vi "Main.vi"() -> ()   [LabVIEW 2020]
doc: "Use this template to build a user interface event handler design pattern. Use this pattern for dialog boxes and other user interfaces. You also can create and execute user-defined events that the VI can handle the same way as user interface events."
uses:
  45491af6-0a4f-43f3-a96b-97e2b64ce829.vi
  87b3b347-8260-4ce2-8b38-5772d22dc736.vi
  421a8988-43c2-4a9a-bdb3-95a91e2f1d3f.vi
  c0ea348c-216c-48f2-902e-4defe1d914fa.vi
  421a8988-43c2-4a9a-bdb3-95a91e2f1d3f.vi/c0db33a9-eb6c-44d9-b982-8563e05d2734.vi
  421a8988-43c2-4a9a-bdb3-95a91e2f1d3f.vi/ae3535a8-0066-4e8d-a5de-b07ac05a7c65.vi
  421a8988-43c2-4a9a-bdb3-95a91e2f1d3f.vi/dda8e586-731b-4197-ad83-6a4d05585a0a.vi
  c0ea348c-216c-48f2-902e-4defe1d914fa.vi/d4db2432-cc9c-482c-8957-dac855435ef6.vi
  c0ea348c-216c-48f2-902e-4defe1d914fa.vi/86fbf154-bd7b-49a2-8ab2-a837b2a95f24.vi
  c0ea348c-216c-48f2-902e-4defe1d914fa.vi/3b95b01e-1ec2-4565-bcd9-7606a5281010.vi
  c0ea348c-216c-48f2-902e-4defe1d914fa.vi/96a08935-737a-44b2-979c-a81d56408f7e.vi
  c0ea348c-216c-48f2-902e-4defe1d914fa.vi/d4db2432-cc9c-482c-8957-dac855435ef6.vi/6eaecd13-6e48-4772-a921-b51ebdf84d88.vi
  c0ea348c-216c-48f2-902e-4defe1d914fa.vi/d4db2432-cc9c-482c-8957-dac855435ef6.vi/d2d5f2b7-06f4-47f6-971c-049c3fdbb653.vi
  c0ea348c-216c-48f2-902e-4defe1d914fa.vi/3b95b01e-1ec2-4565-bcd9-7606a5281010.vi/6eaecd13-6e48-4772-a921-b51ebdf84d88.vi
  c0ea348c-216c-48f2-902e-4defe1d914fa.vi/3b95b01e-1ec2-4565-bcd9-7606a5281010.vi/d2d5f2b7-06f4-47f6-971c-049c3fdbb653.vi
  c0ea348c-216c-48f2-902e-4defe1d914fa.vi/96a08935-737a-44b2-979c-a81d56408f7e.vi/6eaecd13-6e48-4772-a921-b51ebdf84d88.vi
  c0ea348c-216c-48f2-902e-4defe1d914fa.vi/96a08935-737a-44b2-979c-a81d56408f7e.vi/d2d5f2b7-06f4-47f6-971c-049c3fdbb653.vi
  <vilib>/Comparison/Less/Less Functor/Less Functor.lvclass
panel:
  out "Output":string
  in  "Char Pool":string
  in  "Track List":T1(array[cluster])
  in  "stop":bool
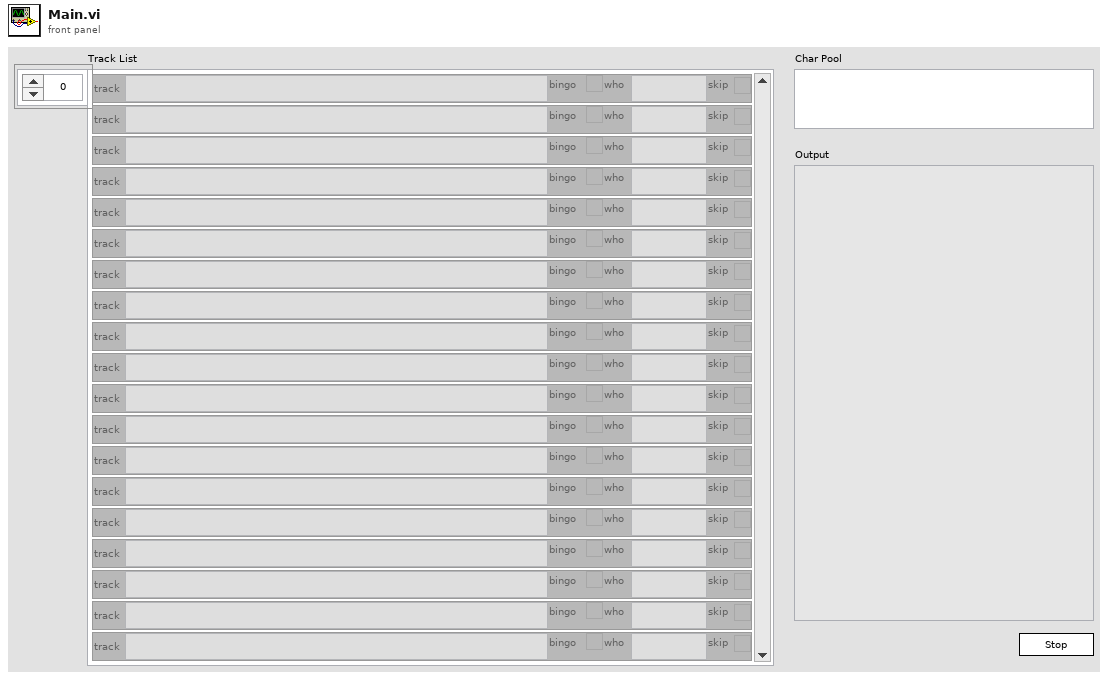
[diagram p1: front panel]
types:
  T1 = cluster{"track":string, "bingo":bool, "who":string, "skip":bool}[]
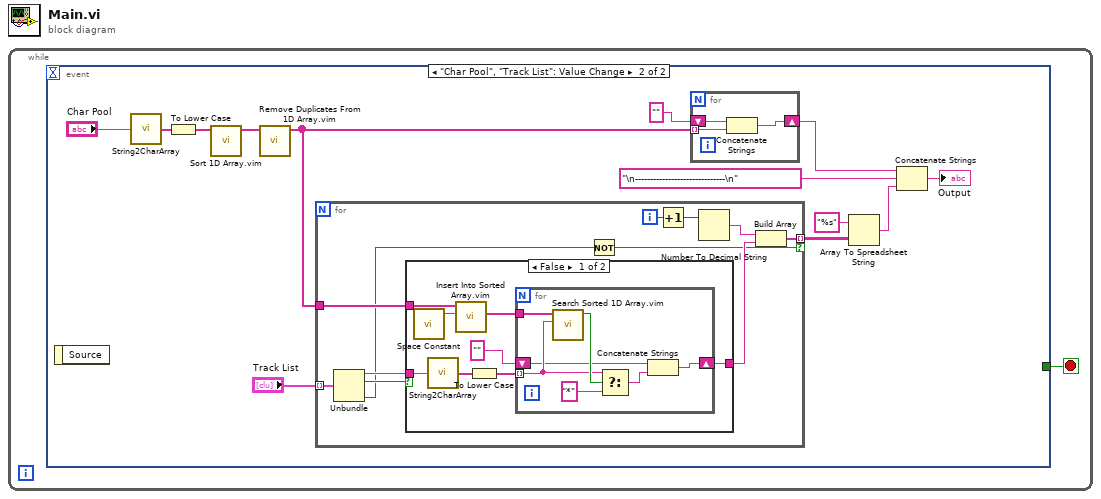
[diagram p0: block diagram]
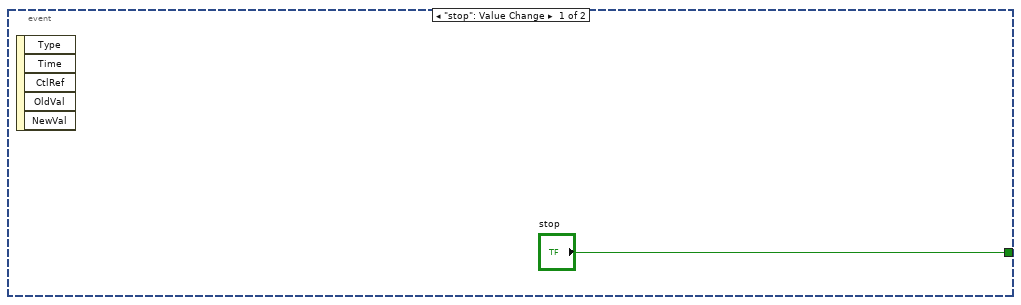
[diagram p2: hidden frame]
diagram:
  n1 = while {
    stop <- w1 stop-if-true
    n2 = event shown="[1] \"Char Pool\", \"Track List\": Value Change" {
      selector: _ -> [_ _]
      dyn-events: _ -> [_ _]
      timeout: _ -> [_ _]
      tunnel: ["stop" _] -> w1
      event "stop": Value Change {
        n3 = event-data() -> ()  [unwired: 1 in, 5 out]
      }
      event "Char Pool", "Track List": Value Change {
        n4 = event-data() -> ()  [unwired: 1 in, 1 out]
        n5 = call "String2CharArray.vi"("String In"="Char Pool") -> ("Char Array"=w7:string[])  [unwired: 4 in]
        n6 = To Lower Case(string=w7) -> (all lower case string=w5:string[])
        n7 = call "Sort 1D Array.vim"("unsorted array"=w5) -> ("sorted array"=w15:string[])  [unwired: 10 in]
        n8 = call "Remove Duplicates From 1D Array.vim"("array"=w15) -> ("array with duplicates removed"=w8:string[])  [unwired: 10 in]
        n9 = for {
          tunnel: "Track List" -> [w25] mode=indexing
          tunnel: [w22] -> w3 mode=indexing if=w16
          tunnel: w8 -> [w18]
          i -> [w26]
          n10 = Unbundle(w25) -> ("track"=w20:string, "bingo"=w21:bool, "skip"=w17:bool)  [unwired: 1 out]
          n11 = case shown="False" w21 {
            tunnel: w20 -> [w33 w42]
            tunnel: [w34 w42] -> w19
            tunnel: w18 -> [w29 _]
            frame False {
              n12 = call <vilib>:"Space Constant.vi"() -> ("String"=w28:string)
              n13 = call "String2CharArray.vi"("String In"=w33) -> ("Char Array"=w32:string[])  [unwired: 4 in]
              n14 = call "Insert Into Sorted Array.vim"("element"=w28, "sorted array in"=w29) -> ("sorted array out"=w30:string[])  [unwired: 9 in]
              n15 = To Lower Case(string=w32) -> (all lower case string=w31:string[])
              n16 = for {
                shift-right: [w36] -> w34
                shift-left: "" ("f") -> [w35]
                tunnel: w30 -> [w40]
                tunnel: w31 -> [w37] mode=indexing
                n17 = call "Search Sorted 1D Array.vim"("element"=w37, "sorted 1D array"=w40) -> ("found?"=w39:bool)  [unwired: 8 in, 1 out]
                n18 = Select(t=w37, s=w39, f="*") -> (s? t:f=w41:string)
                n19 = Concatenate Strings(w35, w41) -> (w36:string)
              }
            }
            frame True {
            }
          }
          n20 = Not(x=w17) -> (.not. x?=w16:bool)
          n21 = Increment(x=w26) -> (x+1=w24:i32)
          n22 = Number To Decimal String(number=w24) -> (decimal integer string=w23:string)  [unwired: 1 in]
          n23 = Build Array(w23, w19) -> (w22:string[])
        }
        n24 = for {
          tunnel: w8 -> [w45] mode=indexing
          shift-right: [w43] -> w13
          shift-left: "" ("string") -> [w44]
          n25 = Concatenate Strings(w44, w45) -> (w43:string)
        }
        n26 = Array To Spreadsheet String(array=w3, 3:"%s" ("format string")) -> (spreadsheet string=w10:string)  [unwired: 1 in]
        n27 = Concatenate Strings(w13, "\n------------------------------\n" ("string"), w10) -> (→"Output":string)
      }
    }
  }
